vi "ClearIfEmpty.vi"(11 "Array":string[](array[string])) -> (3 "ArrayOut":string[](array[string]))   [LabVIEW 2014]
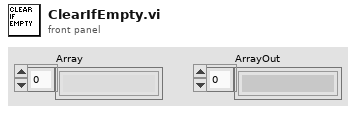
[diagram p1: front panel]
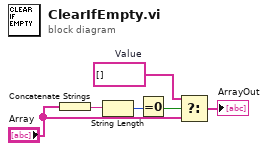
[diagram p0: block diagram]
diagram:
  w4 = string[] []  # Value
  n1 = Concatenate Strings("Array") -> (w1:string)
  n2 = String Length(string=w1) -> (length=w3:i32)
  n3 = Equal To 0?(x=w3) -> (x = 0?=w2:bool)
  n4 = Select(t=w4, s=w2, f="Array") -> (s? t:f=→"ArrayOut":string[])
